vi "dosimat876_run_method.vi"(2 "error in":errorcluster, 3 "Method":string="XDOS1000", 4 "Dosimat Port In":refnum<visa-resource-name>="COM1") -> (0 "error out":errorcluster, 1 "Dosimat Port Out":refnum<visa-resource-name>="COM1")   [LabVIEW 2010]
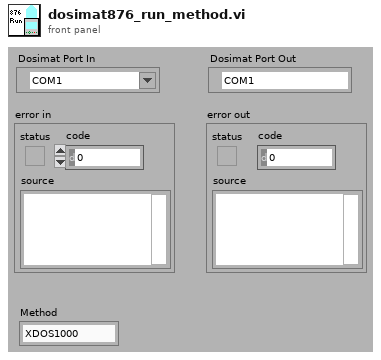
[diagram p1: front panel]
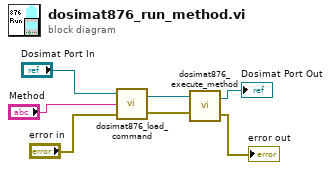
[diagram p0: block diagram]
diagram:
  n1 = call "dosimat876_load_command.vi"("error in"="error in", "Method"="Method", "Dosimat Port In"="Dosimat Port In") -> ("error out"=w3:errorcluster, "Dosimat Port Out"=w4:refnum<visa-resource-name>)
  n2 = call "dosimat876_execute_method.vi"("error in"=w3, "Dosimat Port In"=w4) -> ("error out"=→"error out":errorcluster, "Dosimat Port Out"=→"Dosimat Port Out":refnum<visa-resource-name>)
